vi "Init BLRL Source.vi"(8 "error in (no error)":errorcluster, 10 "Config JSON":string, 11 "BluelinesRedlines Source in":refnum<class "BluelinesRedlines Source.lvclass">) -> (0 "error out":errorcluster, 3 "BluelinesRedlines Source out":refnum<class "BluelinesRedlines Source.lvclass">)   [LabVIEW 2020, in "VolatusGUI.lvlib" / "BluelinesRedlines Source.lvclass"]
uses:
  BluelinesRedlines Source.lvclass
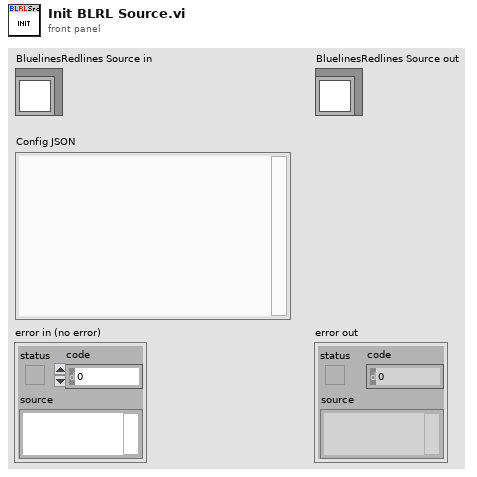
[diagram p1: front panel]
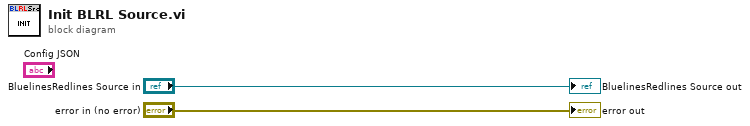
[diagram p0: block diagram]
diagram:
  "error out" <- "error in (no error)"
  "BluelinesRedlines Source out" <- "BluelinesRedlines Source in"
